vi "camera0.vi"() -> ()   [LabVIEW 2015]
uses:
  <vilib>/vision/Image Controls.llb/IMAQ Image.ctl
  <vilib>/userdefined/High Color/IMAQdx.ctl
  <vilib>/vision/driver/NI_Vision_Acquisition_Software.lvlib
panel:
  in  "Cancel Button":bool
  out "Image":T1
  out "appended array":i32[](array[numeric])
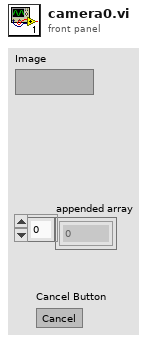
[diagram p1: front panel]
types:
  T1 = typedef "IMAQ Image.ctl" = refnum<image>
  T2 = typedef "IMAQdx.ctl" = refnum<k21>
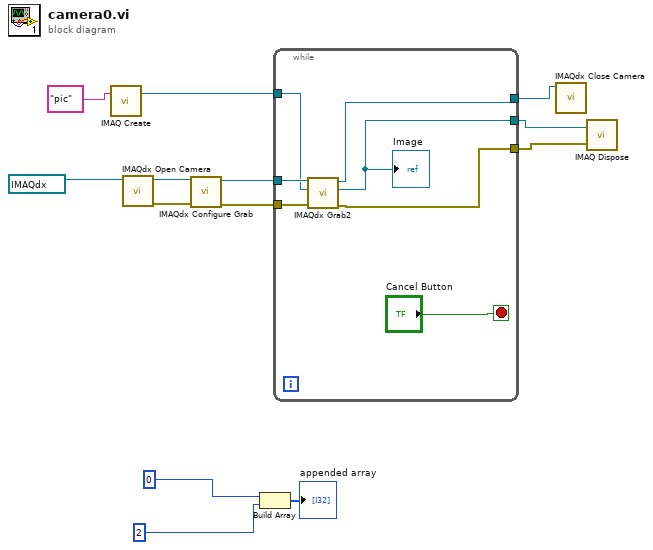
[diagram p0: block diagram]
diagram:
  n1 = call "IMAQ Create"("Image Name"="pic") -> ("New Image"=w5:T1)  [unwired: 4 in, 1 out]
  n2 = call <vilib>:"IMAQdx Open Camera.vi"("Session In"=T2 "cam0" ("IMAQdx Session")) -> ("error out"=w12:errorcluster, "Session Out"=w11:T2)  [unwired: 9 in]
  n3 = call <vilib>:"IMAQdx Configure Grab.vi"("error in"=w12, "Session In"=w11) -> ("error out"=w10:errorcluster, "Session Out"=w9:T2)  [unwired: 8 in]
  n4 = Build Array(0, 2) -> (→"appended array":i32[])
  n5 = while {
    tunnel: w10 -> [w20]
    tunnel: w9 -> [w19]
    tunnel: w5 -> [w18]
    tunnel: [w17] -> w3
    tunnel: [w14] -> w2
    tunnel: [w15] -> w1
    stop <- "Cancel Button" stop-if-true
    n6 = call <vilib>:"IMAQdx Grab2.vi"("error in"=w20, "Image In"=w18, "Session In"=w19) -> ("error out"=w15:errorcluster, "Image Out"=w14:T1, "Session Out"=w17:T2)  [unwired: 5 in, 1 out]
    "Image" <- w14
  }
  n7 = call <vilib>:"IMAQdx Close Camera.vi"("Session In"=w3) -> ()  [unwired: 10 in, 1 out]
  n8 = call "IMAQ Dispose"("Image"=w2, "error in (no error)"=w1) -> ()  [unwired: 4 in, 1 out]
